vi "PT1_discrete.vi"(0 "T":dbl format="%#_13g", 1 "Tcyc":dbl, 2 "AI1":dbl, 3 "Operation":enum16{"Lag", "rapid adjustment"}(ring), 4 "Gain":dbl format="%#_13g", 5 "error in":errorcluster) -> (16 "AO1":dbl, 19 "error out":errorcluster)   [LabVIEW 2022 SP3]
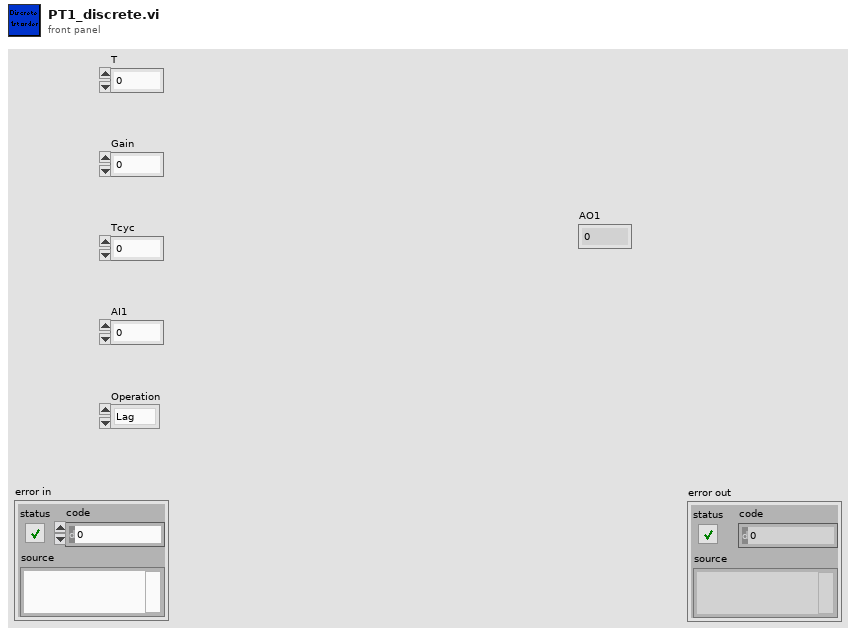
[diagram p1: front panel]
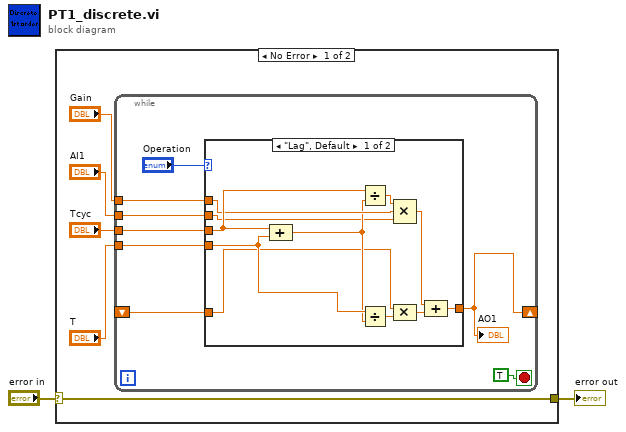
[diagram p0: block diagram]
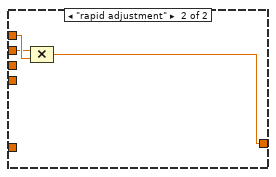
[diagram p2: hidden frame]
diagram:
  n1 = case shown="No Error" "error in" {
    selector: "error in" -> [w3 w30]
    tunnel: [w3 w30] -> w1
    frame No Error {
      n2 = while {
        tunnel: "Tcyc" -> [w13]
        tunnel: "T" -> [w12]
        tunnel: "Gain" -> [w11]
        shift-right: [w8] -> _
        shift-left: _ -> [w9]
        tunnel: "AI1" -> [w10]
        stop <- TRUE stop-if-true
        n3 = case shown="\"Lag\", Default" "Operation" {
          tunnel: w13 -> [w26 _]
          tunnel: w12 -> [w23 _]
          tunnel: w11 -> [w24 w29]
          tunnel: w10 -> [w20 w28]
          tunnel: [w17 w27] -> w8
          tunnel: w9 -> [w16 _]
          frame "Lag", Default {
            n4 = Compound Arithmetic op=ADD(w26, w23) -> (w22:dbl)
            n5 = Divide(x=w26, y=w22) -> (x/y=w25:dbl)
            n6 = Divide(x=w23, y=w22) -> (x/y=w21:dbl)
            n7 = Compound Arithmetic op=MULTIPLY(w25, w24, w20) -> (w19:dbl)
            n8 = Compound Arithmetic op=MULTIPLY(w16, w21) -> (w18:dbl)
            n9 = Compound Arithmetic op=ADD(w19, w18) -> (w17:dbl)
          }
          frame "rapid adjustment" {
            n10 = Compound Arithmetic op=MULTIPLY(w28, w29) -> (w27:dbl)
          }
        }
        "AO1" <- w8
      }
    }
    frame Error {
    }
  }
  "error out" <- w1
